vi "Add Widget to Container.vi"(5 "Container":refnum<class "QWidget.lvclass">, 8 "Error In":errorcluster, 9 "Label":string, 10 "Widget":refnum<class "QWidget.lvclass">, 11 "Splitter Builder in":refnum<class "Splitter Builder.lvclass">) -> (0 "Error Out":errorcluster, 3 "Splitter Builder out":refnum<class "Splitter Builder.lvclass">)   [LabVIEW 2014, in "Splitter Builder.lvclass"]
doc: "Implements the interface provided by Abstract Widget Builder.\n\n\nCopyright (c) 2019 Sze Howe Koh.\nThis code is licensed under the MIT license."
uses:
  Splitter Builder.lvclass
  <vilib>/addons/LQ/Qt Widgets/QWidget/QWidget.lvclass
  <vilib>/addons/LQ/Qt Widgets/QSplitter/QSplitter.lvclass
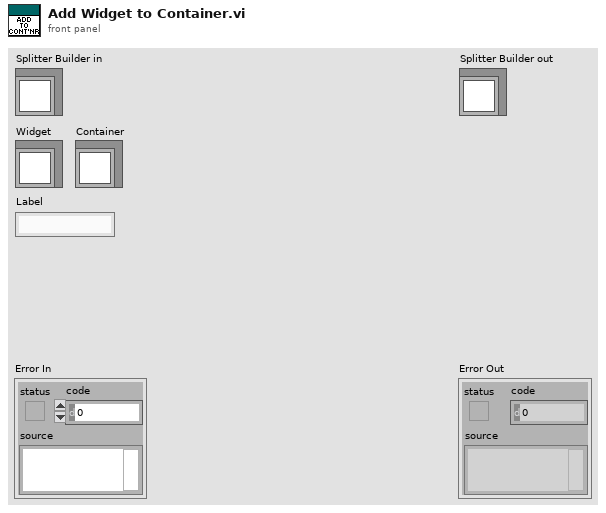
[diagram p1: front panel]
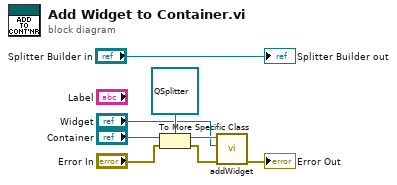
[diagram p0: block diagram]
diagram:
  n1 = To More Specific Class(target class=refnum<class "QSplitter.lvclass"> refnum ("QSplitter"), reference="Container", error in="Error In") -> (specific class reference=w3:refnum<class "QSplitter.lvclass">, error out=w4:errorcluster)
  n2 = call <vilib>:"addWidget.vi"("Error In"=w4, "widget"="Widget", "QSplitter In"=w3) -> ("Error Out"=→"Error Out":errorcluster)  [unwired: 7 in, 1 out]
  "Splitter Builder out" <- "Splitter Builder in"
